vi "Untitled 2.vi"() -> ()   [LabVIEW 2021, in "A3200.lvclass"]
uses:
  A3200.lvclass
  A3200.lvclass/A3200.ctl
  Drivers/Aerotech A3200/Aerotech.lvlib
panel:
  out "Instructions":string
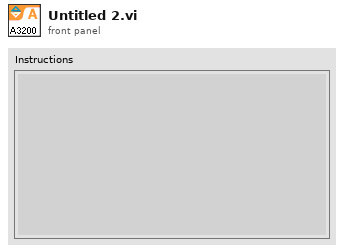
[diagram p1: front panel]
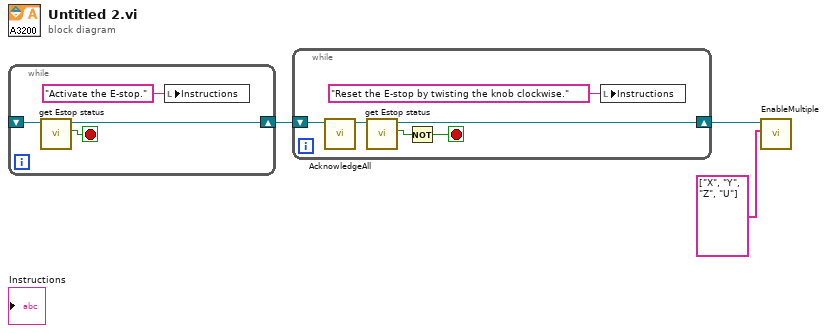
[diagram p0: block diagram]
diagram:
  n1 = while {
    shift-right: [w6] -> w3
    shift-left: _ -> [w7]
    stop <- w5 stop-if-true
    n2 = call "get Estop status.vi"("controller in"=w7) -> ("Estop?"=w5:bool, "controller out"=w6:refnum<k24>)  [unwired: 8 in, 1 out]
    n3 = local write "Instructions"("Activate the E-stop." ("Instructions")) -> ()
  }
  n4 = while {
    shift-right: [w9] -> w1
    shift-left: w3 -> [w11]
    stop <- w12 stop-if-true
    n5 = call "AcknowledgeAll.vi"("controller in"=w11) -> ("controller out"=w10:refnum<k24>)  [unwired: 9 in, 1 out]
    n6 = call "get Estop status.vi"("controller in"=w10) -> ("Estop?"=w13:bool, "controller out"=w9:refnum<k24>)  [unwired: 8 in, 1 out]
    n7 = Not(x=w13) -> (.not. x?=w12:bool)
    n8 = local write "Instructions"("Reset the E-stop by twisting the knob clockwise." ("Instructions")) -> ()
  }
  n9 = call "EnableMultiple.vi"("axis names"=string[] ["X", "Y", "Z", "U"], "controller in"=w1) -> ()  [unwired: 8 in, 2 out]
